vi "PickEvent.vi"(7 "error in (no error)":errorcluster, 10 "CRLF":bool, 11 "Handle In":u64[](array[numeric])) -> (1 "Text":string, 2 "Picked":bool, 3 "Handle Out":u64[](array[numeric]), 5 "error out":errorcluster)   [LabVIEW 2020, in "SnapMB.lvlib"]
uses:
  SnapMB.lvlib
  windows/snapmb.dll
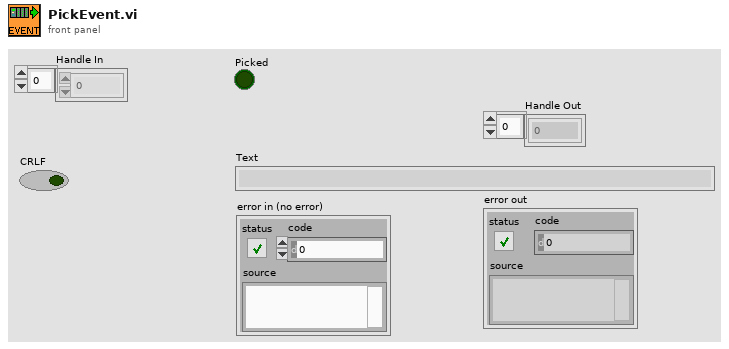
[diagram p1: front panel]
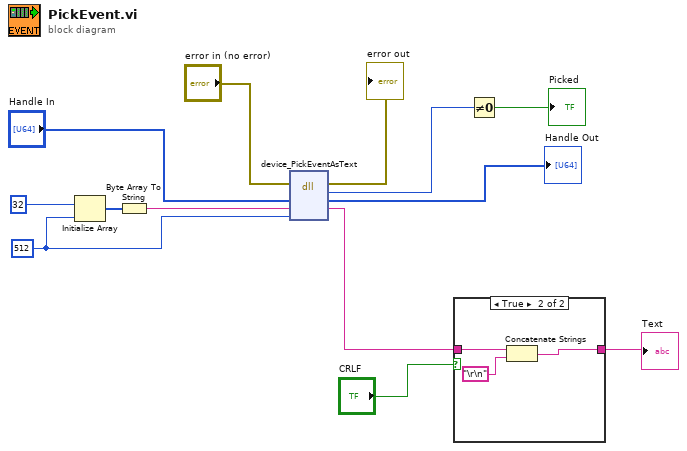
[diagram p0: block diagram]
diagram:
  w10 = 512 ("Dimension Size")
  n1 = Initialize Array(u8 32 ("Element Data"), w10) -> (w13:u8[])
  n2 = Byte Array To String(unsigned byte array=w13) -> (string=w11:string)
  n3 = dll-call lib="D:/SnapMB/LabView/lib/windows/snapmb.dll" fn="device_PickEventAsText"(error in="error in (no error)", "Device"="Handle In", "Text"=w11, "TextSize"=w10) -> (error out=→"error out":errorcluster, "Result"=w8:i32, "Device"=→"Handle Out":u64[], "Text"=w4:string)  [unwired: 3 in, 1 out]
  n4 = case shown="True" "CRLF" {
    tunnel: w4 -> [w14 w16]
    tunnel: [w14 w15] -> w3
    frame False {
    }
    frame True {
      n5 = Concatenate Strings(w16, "\r\n") -> (w15:string)
    }
  }
  "Text" <- w3
  n6 = Not Equal To 0?(x=w8) -> (x != 0?=→"Picked":bool)
